vi "Write Table To Excel.vi"(0 "Table":string[][](table)=[["1", "2", "3", "4", "5", "6", "7", "8", "9", "10"], ["10", "11", "12", "13", "14", "15", "16", "17", "18", "19"], ["20", "21", "22", "23", "24", "25", "26", "27", "28", "29"], ["30", "31", "32", "33", "34", "35", "36", "37", "38", "39"]], 2 "Filename":string="c:\\file", 4 "Completion Task":u16(ring) items=["Leave Excel Open", "Close Spreadsheet"]) -> ()   [LabVIEW 2010]
doc: "This VI demonstrates the basic idea of using the OLE Automation VIs by writing a Table into an Excel WorkSheet."
panel:
  out "error out":errorcluster
  in  "error in (no error)":errorcluster
  # "This VI demostrates the basic steps needed to enter the values in a table into a spreadsheet and then save it to a file."
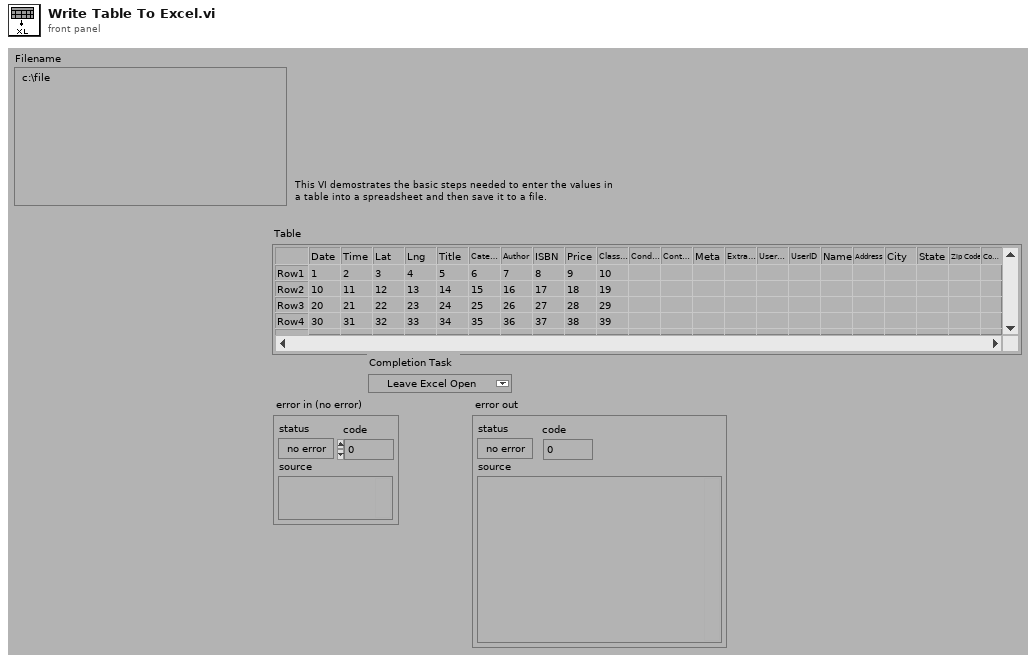
[diagram p1: front panel]
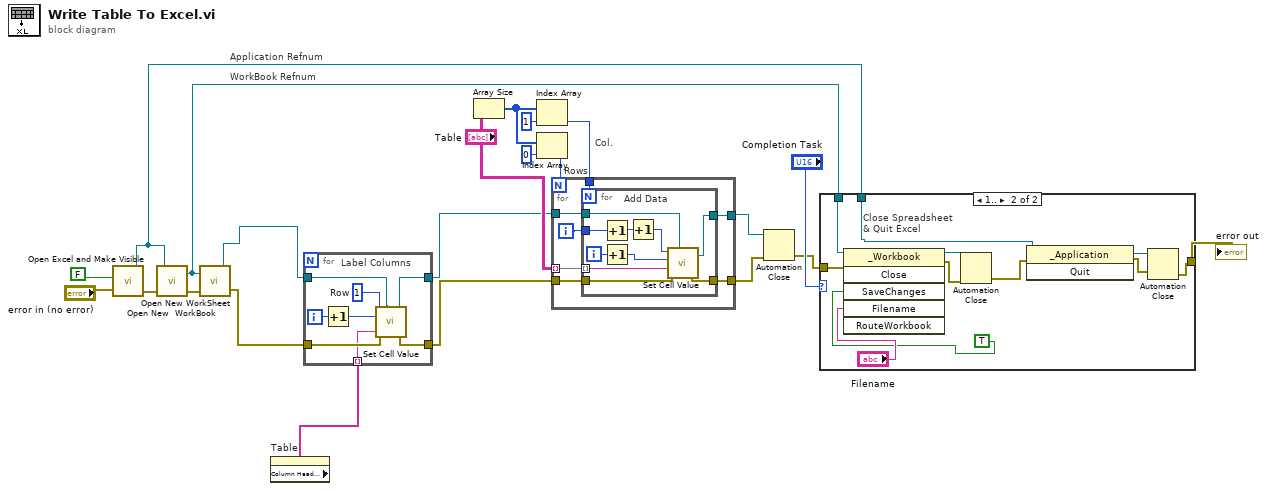
[diagram p0: block diagram]
diagram:
  # "Col."
  # "Rows"
  # "WorkBook Refnum"
  # "Application Refnum"
  n1 = call "Open Excel and Make Visible.vi"("error in (no error)"="error in (no error)", "Visible Boolean"=FALSE) -> ("error out"=w17:errorcluster, "Excel._Application"=w10:refnum<k7>)
  n2 = call "Open New  WorkBook.vi"("error in (no error)"=w17, "Excel._Application"=w10) -> ("error out"=w16:errorcluster, "Excel._Workbook"=w11:refnum<k7>)  [unwired: 1 out]
  n3 = call "Open New WorkSheet.vi"("error in (no error)"=w16, "Excel._Workbook"=w11) -> ("error out"=w5:errorcluster, "Excel._Worksheet"=w3:refnum<k7>)  [unwired: 1 out]
  n4 = property on="Table" class="Tbl (strict)"() -> ("Column Header Strings[]"=w1:string[])  [unwired: 2 in, 2 out]
  n5 = for {
    tunnel: w3 -> [w29]
    tunnel: w5 -> [w28]
    tunnel: [w27] -> w4
    tunnel: [w26] -> w2
    tunnel: w1 -> [w24] mode=indexing
    i -> [w30]
    w25 = 1  # Row
    # "Label Columns"
    n6 = Increment(x=w30) -> (x+1=w23:i32)
    n7 = call "Set Cell Value.vi"("Row"=w25, "Col"=w23, "Value"=w24, "error in (no error)"=w28, "Excel._Worksheet"=w29) -> ("Excel._Worksheet"=w26:refnum<k7>, "error out"=w27:errorcluster)
  }
  n8 = Array Size(array="Table") -> (size(s)=w22:i32[])
  n9 = Index Array(array=w22, index=1) -> (element=w14:i32)
  n10 = Index Array(array=w22, index=0) -> (element=w13:i32)
  n11 = for {
    N: w13 -> [_]
    tunnel: w2 -> [w37]
    tunnel: w4 -> [w34]
    tunnel: [w36] -> w8
    tunnel: "Table" -> [w33] mode=indexing
    tunnel: w14 -> [w32]
    tunnel: [w31] -> w6
    i -> [w35]
    n12 = for {
      N: w32 -> [_]
      tunnel: w37 -> [w46]
      tunnel: w34 -> [w45]
      tunnel: [w44] -> w36
      tunnel: w35 -> [w43]
      tunnel: w33 -> [w42] mode=indexing
      tunnel: [w41] -> w31
      i -> [w47]
      # "Add Data"
      n13 = Increment(x=w43) -> (x+1=w39:i32)
      n14 = Increment(x=w47) -> (x+1=w40:i32)
      n15 = Increment(x=w39) -> (x+1=w38:i32)
      n16 = call "Set Cell Value.vi"("Row"=w38, "Col"=w40, "Value"=w42, "error in (no error)"=w45, "Excel._Worksheet"=w46) -> ("Excel._Worksheet"=w41:refnum<k7>, "error out"=w44:errorcluster)
    }
  }
  n17 = Automation Close(3:w8, 5:w6) -> (0:w7:errorcluster)
  n18 = case shown="1.." "Completion Task" {
    tunnel: [w48 w51] -> w9
    tunnel: w11 -> [_ w59]
    tunnel: w10 -> [_ w55]
    tunnel: w7 -> [w48 w58]
    frame ..0 {
    }
    frame 1.. {
      # "Close Spreadsheet\n& Quit Excel"
      n19 = invoke class="_Workbook" method="Close"(reference=w59, error in=w58, "SaveChanges"=TRUE, "Filename"="Filename") -> (reference out=w57:refnum<k7>, error out=w56:errorcluster)  [unwired: 2 in, 4 out]
      n20 = Automation Close(3:w56, 5:w57) -> (0:w54:errorcluster)
      n21 = invoke class="_Application" method="Quit"(reference=w55, error in=w54) -> (reference out=w52:refnum<k7>, error out=w53:errorcluster)  [unwired: 1 in, 1 out]
      n22 = Automation Close(3:w53, 5:w52) -> (0:w51:errorcluster)
    }
  }
  "error out" <- w9
